vi "Append Space.vi"(1 "INPUT STRING":string) -> (0 "OUTPUT STRING (PLUS [SPACE])":string)   [LabVIEW 2019]
doc: "Concatenates a SPACE [ ] at the end of the input string. Copyright Laouris & Reinking, May 89"
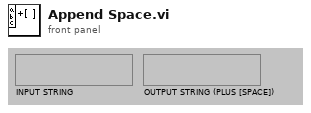
[diagram p1: front panel]
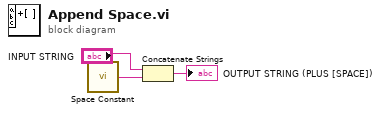
[diagram p0: block diagram]
diagram:
  n1 = call <vilib>:"Space Constant.vi"() -> ("String"=w3:string)
  n2 = Concatenate Strings("INPUT STRING", w3) -> (→"OUTPUT STRING (PLUS [SPACE])":string)
